vi "Transmit.vi"(6 "VCI_CAN_OBJ":T1={"ID"=4657, "TimeStamp"=0, "TimeFlag"=0, "SendType"=0, "RemoteFlag"=0, "ExternFlag"=0, "DataLen"=0, "Data"=0, 0, 0, 0, 0, 0, 0, 0, "Reserved"=0, 0, 0} {"ID" format="%x"}, 8 "Len":u32=8, 9 "CANIndex":u32, 10 "DevIndex":u32, 11 "DevType":u32) -> (1 "CANIndex 2":u32, 2 "DevIndex 2":u32, 3 "DevType 2":u32, 5 "sendNUM":i32=1)   [LabVIEW 2016]
uses:
  ECanVci.dll
panel:
  out "Len 2":u32=1
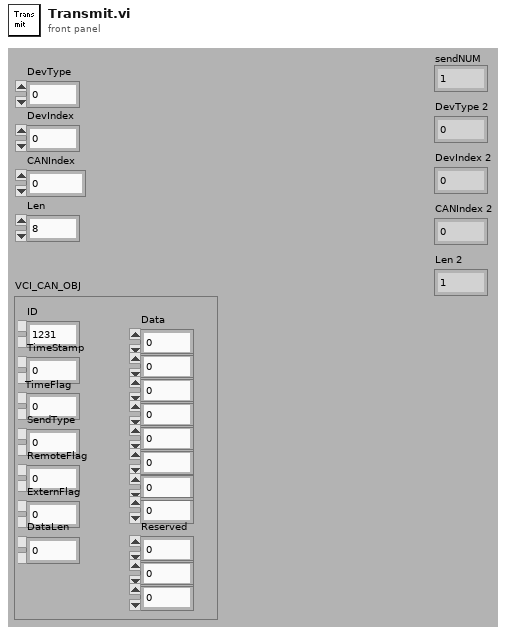
[diagram p1: front panel]
types:
  T1 = cluster{"ID":u32, "TimeStamp":u32, "TimeFlag":u8, "SendType":u8, "RemoteFlag":u8, "ExternFlag":u8, "DataLen":u8, "Data":u8, u8, u8, u8, u8, u8, u8, u8, "Reserved":u8, u8, u8}
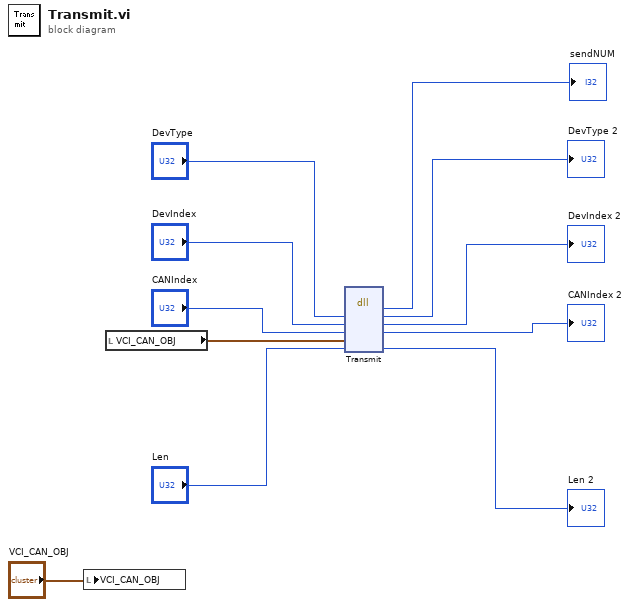
[diagram p0: block diagram]
diagram:
  n1 = local write "VCI_CAN_OBJ"("VCI_CAN_OBJ") -> ()
  n2 = local read "VCI_CAN_OBJ"() -> (w2:T1)
  n3 = dll-call lib="C:/Users/Azmat/Desktop/Labview/ECanVci.dll" fn="Transmit"("DevType"="DevType", "DevIndex"="DevIndex", "CANIndex"="CANIndex", "CAN_OBJ"=w2, "Len"="Len") -> ("sendNUM"=→"sendNUM":i32, "DevType"=→"DevType 2":u32, "DevIndex"=→"DevIndex 2":u32, "CANIndex"=→"CANIndex 2":u32, "Len"=→"Len 2":u32)  [unwired: 4 in, 2 out]
